vi "Basic Operations.vi"() -> ()   [LabVIEW 2019, in "Tree Map.lvlib"]
doc: "<b>Author:</b> Piotr Kruczkowski <PrimaryKey>\n<b>License:</b> NewBSD\n\nCopyright (c) 2019, National Instruments\nAll rights reserved.\n\nRedistribution and use in source and binary forms, with or without\nmodification, are permitted provided that the following conditions are met:\n1. Redistributions of source code must retain the above copyright\n notice, this list of conditions and the following disclaimer.\n2. Redistributions in binary form must reproduce the above copyright\n notice, this list of conditions and the following disclaimer in the\n documentation and/or other materials provided with the distribution.\n3. Neither the name of National Instruments nor the\n names of its contributors may be used to endorse or promote products\n derived from this software without specific prior written permission.\n\nTHIS SOFTWARE IS PROVIDED BY National Instruments ''AS IS'' AND ANY\nEXPRESS OR IMPLIED WARRANTIES, INCLUDING, BUT NOT LIMITED TO, THE IMPLIED\nWARRANTIES OF MERCHANTABILITY AND FITNESS FOR A PARTICULAR PURPOSE ARE\nDISCLAIMED. IN NO EVENT SHALL National Instruments BE LIABLE FOR ANY\nDIRECT, INDIRECT, INCIDENTAL, SPECIAL, EXEMPLARY, OR CONSEQUENTIAL DAMAGES\n(INCLUDING, BUT NOT LIMITED TO, PROCUREMENT OF SUBSTITUTE GOODS OR SERVICES;\nLOSS OF USE, DATA, OR PROFITS; OR BUSINESS INTERRUPTION) HOWEVER CAUSED AND\nON ANY THEORY OF LIABILITY, WHETHER IN CONTRACT, STRICT LIABILITY, OR TORT\n(INCLUDING NEGLIGENCE OR OTHERWISE) ARISING IN ANY WAY OUT OF THE USE OF THIS\nSOFTWARE, EVEN IF ADVISED OF THE POSSIBILITY OF SUCH DAMAGE."
uses:
  Tree Map.lvlib
  Utility/Into Tree Control Items.vi
panel:
  out "Root Paths Set":set{string}(c389)={"\\Base"}
  out "size":i32=3
  out "empty?":bool=TRUE
  in  "Tree Control":string(tree)
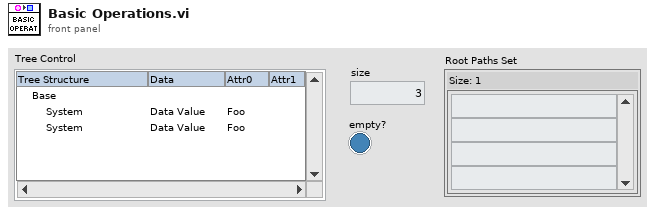
[diagram p1: front panel]
types:
  T1 = typedef "Tree Map.lvlib/Tree Map Data.ctl" = map{string, cluster{"Child Paths Set":set{string}, "Name":string, "Data":string, "Attributes":map{string, string}}}
  T2 = cluster{"Left Cell String":string, "Child Text":string[], "Child Tag":string, "Item Indent":i32, "Child Only?":bool, "Glyph Index":i32}[]
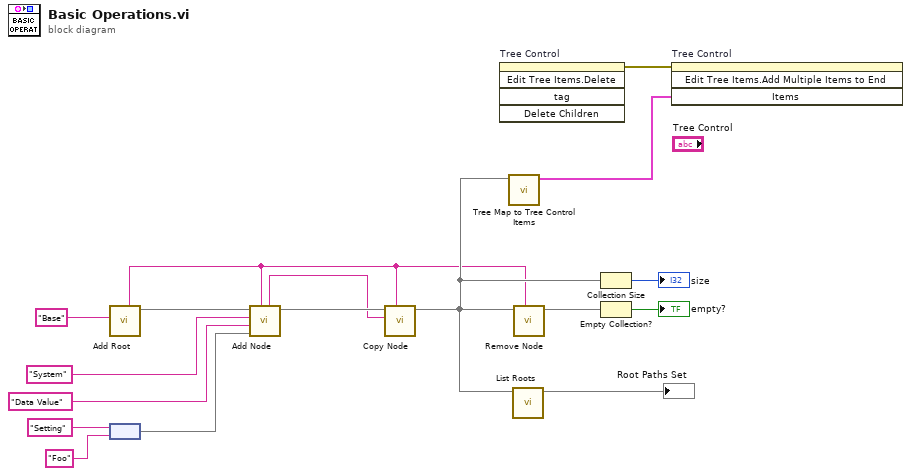
[diagram p0: block diagram]
diagram:
  n1 = call "Add Root.vi"("New Root Name"="Base") -> ("Tree Map Out"=w15:T1, "Root Path"=w3:string)  [unwired: 9 in]
  n2 = node("Setting" ("New Root Name"), "Foo" ("New Root Name")) -> (w12:map{string, string})
  n3 = call "Add Node.vi"("Parent Path"=w3, "Attributes"=w12, "Data"="Data Value" ("New Root Name"), "New Node Name"="System" ("New Root Name"), "Tree Map In"=w15) -> ("Tree Map Out"=w2:T1, "New Node Path"=w1:string)  [unwired: 4 in, 1 out]
  n4 = call "Copy Node.vi"("New Parent Path in Target"=w3, "Node Path in Source"=w1, "Target Tree Map In"=w2) -> ("Target Tree Map Out"=w5:T1)  [unwired: 6 in, 2 out]
  n5 = invoke on="Tree Control" class="Tree (strict)" method="Edit Tree Items.Delete"() -> (error out=w17:errorcluster)  [unwired: 5 in, 4 out]
  n6 = call "Tree Map to Tree Control Items.vi"("Tree Map In"=w5) -> ("Tree Control Items"=w6:T2)  [unwired: 10 in]
  n7 = call "List Roots.vi"("Tree Map In"=w5) -> ("Unique Root Paths Set"=→"Root Paths Set":set{string})  [unwired: 10 in]
  n8 = call "Remove Node.vi"("Node Path"=w3, "Tree Map In"=w5) -> ("Tree Map Out"=w9:T1)  [unwired: 7 in, 2 out]
  n9 = Collection Size(1:w5) -> (0:→"size":i32)
  n10 = Empty Collection?(1:w9) -> (0:→"empty?":bool)
  n11 = invoke on="Tree Control" class="Tree (strict)" method="Edit Tree Items.Add Multiple Items to End"(error in=w17, "Items"=w6) -> ()  [unwired: 2 in, 4 out]
